vi "Voorbeeld_Event_Driven_Programmeren_02_io.vi"() -> ()   [LabVIEW 2019]
panel:
  out "Led":bool
  in  "Schakelaar":bool
  in  "stop":bool
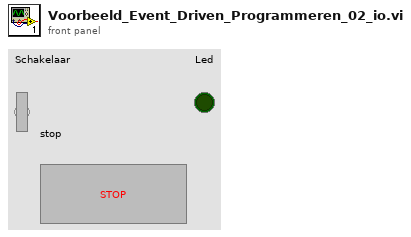
[diagram p1: front panel]
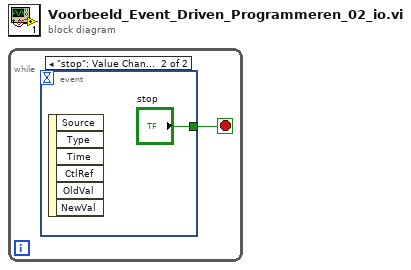
[diagram p0: block diagram]
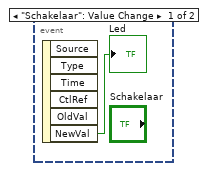
[diagram p2: hidden frame]
diagram:
  n1 = while {
    stop <- w1 stop-if-true
    n2 = event shown="[1] \"stop\": Value Change" {
      selector: _ -> [_ _]
      dyn-events: _ -> [_ _]
      timeout: _ -> [_ _]
      tunnel: [_ "stop"] -> w1
      event "Schakelaar": Value Change {
        n3 = event-data() -> ("NewVal"=→"Led":bool)  [unwired: 1 in, 5 out]
      }
      event "stop": Value Change {
        n4 = event-data() -> ()  [unwired: 1 in, 6 out]
      }
    }
  }
